vi "To String.vi"(8 "error in (no error)":errorcluster, 11 "Double in":refnum<class "Double.lvclass">) -> (0 "error out":errorcluster, 2 "String":string)   [LabVIEW 2020, in "Data.lvlib" / "Double.lvclass"]
doc: "Convert 'Generic Data in' to a string.\nThe default implementation convert the data to an XML string."
uses:
  Double.lvclass
  Double.lvclass/Double.ctl
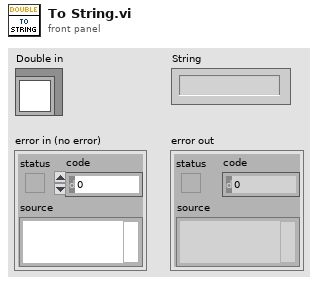
[diagram p1: front panel]
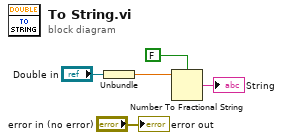
[diagram p0: block diagram]
diagram:
  n1 = Unbundle("Double in") -> (w3:dbl)
  n2 = Number To Fractional String(use system decimal point (T)=FALSE, number=w3) -> (F-format string=→"String":string)  [unwired: 2 in]
  "error out" <- "error in (no error)"
